vi "SendValues.vi"() -> ()   [LabVIEW 2015]
uses:
  <vilib>/httpClient/POSTBuffer.vi
  <vilib>/httpClient/LabVIEWHTTPClient.lvlib
panel:
  out "body":string
  out "headers":string
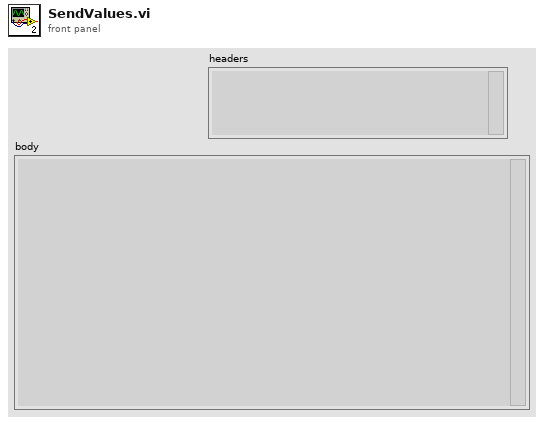
[diagram p1: front panel]
types:
  T1 = typedef "LabVIEWHTTPClient.lvlib/ClientHandle.ctl" = refnum<k1>
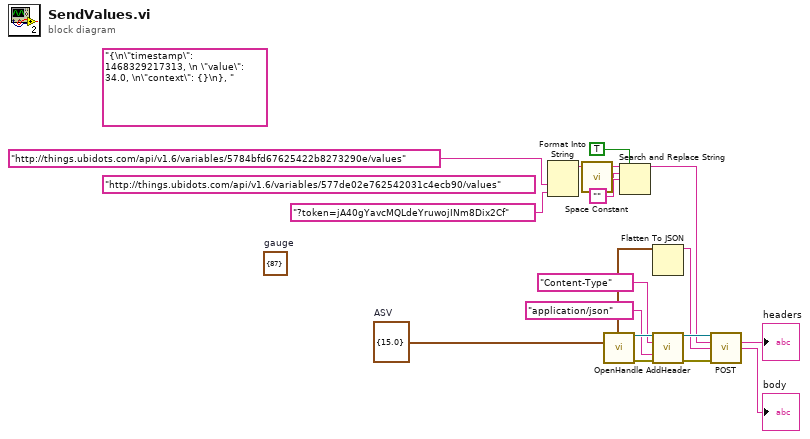
[diagram p0: block diagram]
diagram:
  w2 = cluster{"value":dbl} {"value"=15.0}  # ASV
  (unwired) "http://things.ubidots.com/api/v1.6/variables/577de02e762542031c4ecb90/values"
  (unwired) "{\n\"timestamp\": 1468329217313, \n \"value\": 34.0, \n\"context\": {}\n}, "
  (unwired) cluster{"value":i32} {"value"=87}  # gauge
  n1 = Format Into String("http://things.ubidots.com/api/v1.6/variables/5784bfd67625422b8273290e/values", "?token=jA40gYavcMQLdeYruwojINm8Dix2Cf") -> (resulting string=w4:string)  [unwired: 3 in, 1 out]
  n2 = call <vilib>:"Space Constant.vi"() -> ("String"=w7:string)
  n3 = call <vilib>:"OpenHandle.vi"() -> ("client handle out"=w16:T1, "error out"=w14:errorcluster)  [unwired: 14 in]
  n4 = Search and Replace String(replace all?=TRUE ("replace all? (F)"), input string=w4, search string=w7, replace string="" ("Empty String Constant")) -> (result string=w3:string)  [unwired: 4 in, 3 out]
  n5 = Flatten To JSON(anything=w2) -> (JSON string=w9:string)  [unwired: 2 in, 1 out]
  n6 = call <vilib>:"AddHeader.vi"("client handle"=w16, "header"="Content-Type", "value"="application/json" ("Combo Box"), "error in (no error)"=w14) -> ("client handle out"=w17:T1, "error out"=w15:errorcluster)  [unwired: 10 in]
  n7 = call-poly <vilib>:"POST.vi"("client handle"=w17, "url"=w3, "buffer"=w9, "error in (no error)"=w15) -> ("headers"=→"headers":string, "body"=→"body":string)  [unwired: 8 in, 2 out]
